vi "9-5 2진파일에쓰기.vi"() -> ()   [LabVIEW 2014]
uses:
  <vilib>/Analysis/NI_AALBase.lvlib
panel:
  out "웨이브폼 그래프":dbl[](graph)
  in  "파일 경로(대화 상자 사용)":path=path "C:/Users/LVEDU09/Documents/YSK/2019-03-08/샘플 000.txt"
  out "에러 출력":errorcluster
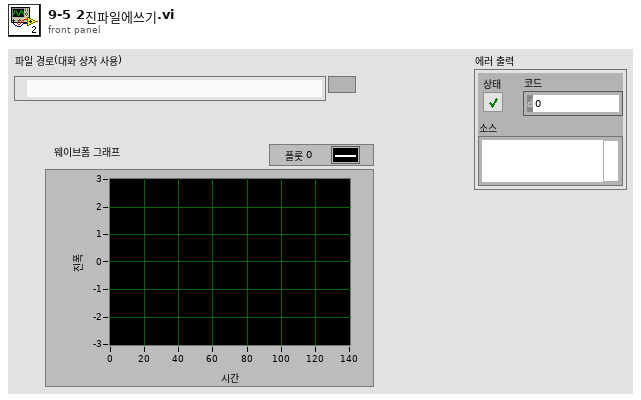
[diagram p1: front panel]
types:
  T1 = enum16{"open", "replace", "create", "open or create", "replace or create", "replace or create with confirmation"}
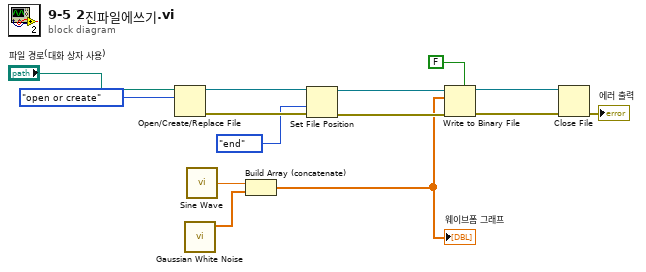
[diagram p0: block diagram]
diagram:
  n1 = Open/Create/Replace File(file path (use dialog)="파일 경로(대화 상자 사용)", operation (0:open)=T1."open or create" ("동작(0:open)")) -> (refnum out=w6:refnum<file>, error out=w5:errorcluster)  [unwired: 4 in, 1 out]
  n2 = call <vilib>:"Gaussian White Noise.vi"() -> ("Gaussian noise pattern"=w7:dbl[])  [unwired: 10 in, 1 out]
  n3 = call <vilib>:"Sine Wave.vi"() -> ("phase out"=w8:dbl)  [unwired: 5 in, 2 out]
  n4 = Build Array (concatenate)(w8, w7) -> (w1:dbl[])
  "웨이브폼 그래프" <- w1
  n5 = Set File Position(refnum=w6, from (0:start)=enum16{"start", "end", "current"}."end" ("시작(0:시작)"), error in=w5) -> (refnum out=w4:refnum<file>, error out=w3:errorcluster)  [unwired: 1 in]
  n6 = Write to Binary File(file (use dialog)=w4, data=w1, error in=w3, 5:FALSE ("배열 또는 문자열 크기를 앞에 추가? (참)")) -> (refnum out=w14:refnum<file>, error out=w13:errorcluster)  [unwired: 2 in, 1 out]
  n7 = Close File(refnum=w14, error in=w13) -> (error out=→"에러 출력":errorcluster)  [unwired: 1 out]
